vi "质控停止子VI.vi"(11 "数组":bool[](array[boolean])) -> ()   [LabVIEW 2016, in "质控单元V1.lvlib"]
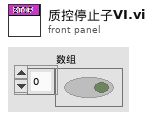
[diagram p1: front panel]
types:
  T1 = enum16{"待机", "水样测试（全流程）", "停止", "加标回收", "水样测试（简易流程）"}
  T2 = typedef "质控单元V1.lvlib/质控slave id.ctl" = enum16{"null", "氨氮", "总磷", "CODMn", "CODCr", "总氮"}
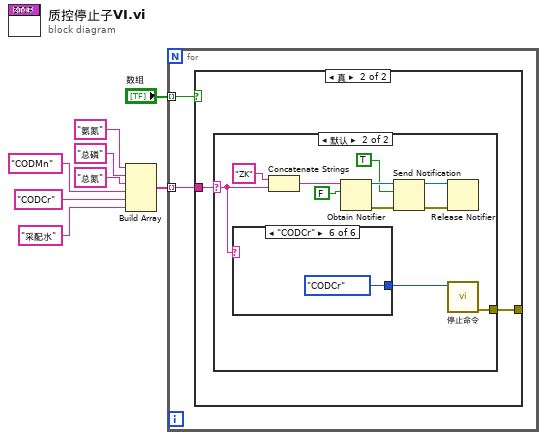
[diagram p0: block diagram]
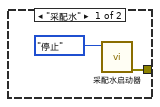
[diagram p3: hidden frame]
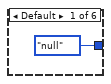
[diagram p4: hidden frame]
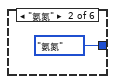
[diagram p5: hidden frame]
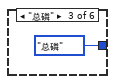
[diagram p6: hidden frame]
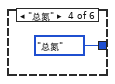
[diagram p7: hidden frame]
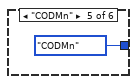
[diagram p8: hidden frame]
diagram:
  n1 = Build Array("氨氮", "总磷", "总氮", "CODMn", "CODCr", "采配水") -> (w6:string[])
  n2 = for {
    tunnel: w6 -> [w10] mode=indexing
    tunnel: "数组" -> [w9] mode=indexing
    n3 = case shown="真" w9 {
      tunnel: w10 -> [_ w11]
      tunnel: [_ w12] -> _
      frame False {
      }
      frame True {
        n4 = case shown="默认" w11 {
          selector: w11 -> [_ w15]
          tunnel: [w14 w16] -> w12
          frame "采配水" {
            n5 = call "采配水启动器.vi"("启动/停止命令"=T1."停止") -> ("error out"=w14:errorcluster)  [unwired: 10 in]
          }
          frame Default {
            n6 = case shown="\"CODCr\"" w15 {
              tunnel: [质控slave_id."null" ("Slave ID") 质控slave_id."氨氮" ("Slave ID") 质控slave_id."总磷" ("Slave ID") 质控slave_id."总氮" ("Slave ID") 质控slave_id."CODMn" ("Slave ID") 质控slave_id."CODCr" ("Slave ID")] -> w17
              frame Default {
              }
              frame "氨氮" {
              }
              frame "总磷" {
              }
              frame "总氮" {
              }
              frame "CODMn" {
              }
              frame "CODCr" {
              }
            }
            n7 = Concatenate Strings("ZK" ("名称（未命名）"), w15) -> (w23:string)
            n8 = Obtain Notifier(name (unnamed)=w23, notification data type=FALSE) -> (notifier out=w22:refnum<notifier>, error out=w21:errorcluster)  [unwired: 2 in, 1 out]
            n9 = Send Notification(notification=TRUE ("通知"), notifier=w22, error in (no error)=w21) -> (notifier out=w20:refnum<notifier>, error out=w19:errorcluster)
            n10 = Release Notifier(notifier=w20, error in (no error)=w19) -> ()  [unwired: 1 in, 3 out]
            n11 = call "停止命令.vi"("Slave ID"=w17) -> ("error out"=w16:errorcluster)  [unwired: 10 in]
          }
        }
      }
    }
  }
